vi "read_attempt.vi"() -> ()   [LabVIEW 2014]
panel:
  out "read buffer":string
  in  "VISA resource name":refnum<visa-resource-name>
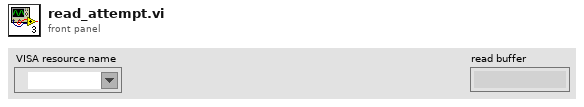
[diagram p1: front panel]
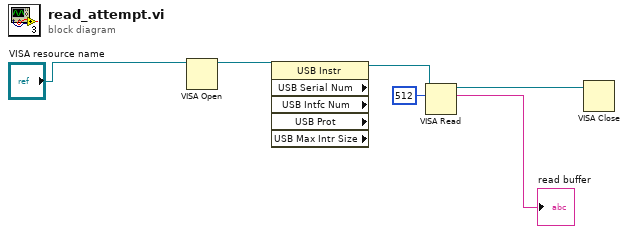
[diagram p0: block diagram]
diagram:
  n1 = VISA Open(VISA resource name="VISA resource name") -> (VISA resource name=w5:refnum<visa-resource-name>)  [unwired: 4 in, 1 out]
  n2 = property class="USB Instr" props=["USB Serial Num", "USB Intfc Num", "USB Prot", "USB Max Intr Size"](reference=w5) -> (reference out=w4:refnum<visa-resource-name>)  [unwired: 1 in, 5 out]
  n3 = VISA Read(VISA resource name=w4, byte count=u32 512) -> (VISA resource name out=w2:refnum<visa-resource-name>, read buffer=→"read buffer":string)  [unwired: 1 in, 2 out]
  n4 = VISA Close(VISA resource name=w2) -> ()  [unwired: 1 in, 1 out]
